vi "setUp.vi"(8 "error in (no error)":errorcluster, 11 "reference in":refnum<class "Disabled Custom Device.lvclass">) -> (0 "error out":errorcluster, 3 "reference out":refnum<class "Disabled Custom Device.lvclass">)   [LabVIEW 2020, in "Disabled Custom Device.lvclass"]
doc: "setUp runs prior to the test method during test execution. Use this method to initialize any object data required by your tests."
uses:
  Disabled Custom Device.lvclass
  C:/Program Files (x86)/National Instruments/LabVIEW 2020/vi.lib/addons/_JKI Toolkits/VI Tester/TestCase.llb/TestCase.lvclass
  Disabled Custom Device.lvclass/Disabled Custom Device.ctl
  <vilib>/addons/_JKI Toolkits/VI Tester/TestCase.llb/TestCase.lvclass
  niveristand-custom-device-testing-tools/VeriStandTestUtilities/VeriStandTestUtilities.lvlib
  Scripting/Ballard/Ballard ARINC 429 Scripting.lvlib
  C:/dev/git/niveristand-custom-device-testing-tools/VeriStandTestCase/VeriStandTestCase.lvclass
  C:/dev/git/niveristand-ballard-arinc429-custom-device/Source/Custom Device Support/Tests/System/Disabled Custom Device/Disabled Custom Device.lvclass
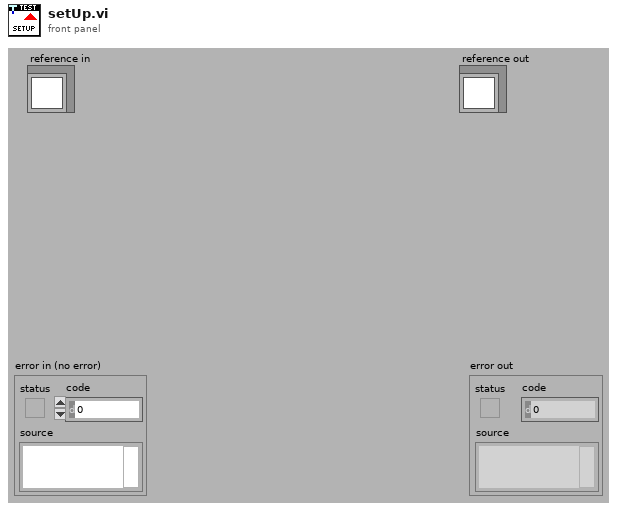
[diagram p1: front panel]
types:
  T1 = typedef "Custom Device API.lvlib/Custom Device Item Ref.ctl" = u64
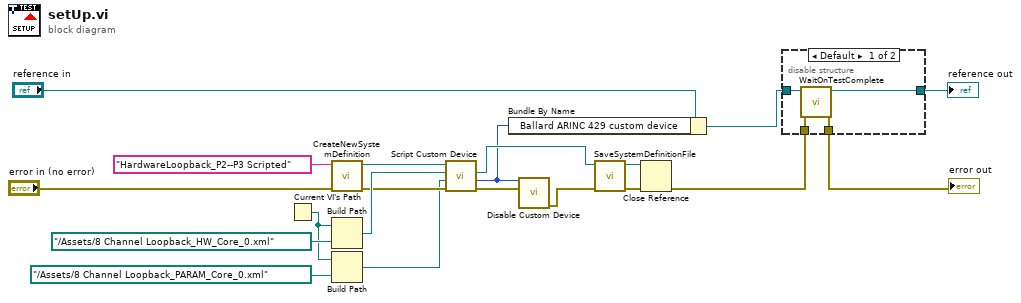
[diagram p0: block diagram]
diagram:
  n1 = Current VI's Path() -> (path=w4:path)
  n2 = call "CreateNewSystemDefinition.vi"("error in"="error in (no error)", "System Definition Name"="HardwareLoopback_P2--P3 Scripted" ("Channel")) -> ("error out"=w13:errorcluster, "System Definition Path"=w12:path)  [unwired: 8 in]
  n3 = Build Path(base path=w4, name or relative path=path "../Assets/8 Channel Loopback_HW_Core_0.xml" ("Hardware File Path")) -> (appended path=w17:path)
  n4 = Build Path(base path=w4, name or relative path=path "../Assets/8 Channel Loopback_PARAM_Core_0.xml" ("Hardware File Path")) -> (appended path=w5:path)
  n5 = call "Script Custom Device.vi"("error in"=w13, "Parameter File Path"=w5, "Hardware File Path"=w17, "System Definition File Path In"=w12) -> ("error out"=w3:errorcluster, "Ballard ARINC 429 custom device out"=w1:T1, "System Definition Reference"=w11:refnum<k24>)  [unwired: 4 in, 1 out]
  n6 = Bundle By Name(cluster="reference in", "Ballard ARINC 429 custom device"=w1) -> (w7:refnum<class "Disabled Custom Device.lvclass">)
  n7 = call "Disable Custom Device.vi"("error in (no error)"=w3, "Ballard ARINC 429 ref"=w1) -> ("error out"=w2:errorcluster)  [unwired: 8 in, 1 out]
  n8 = call "SaveSystemDefinitionFile.vi"("error in (no error)"=w2, "System Definition Reference in"=w11) -> ("error out"=w9:errorcluster, "System Definition Reference out"=w8:refnum<k24>)  [unwired: 8 in]
  n9 = Close Reference(reference=w8, error in (no error)=w9) -> (error out=w6:errorcluster)
  n10 = disable-structure shown="Default" {
    disable-tunnel: w6 -> [w24 w25]
    disable-tunnel: [w23 w25] -> w20
    disable-tunnel: [w22 w26] -> w18
    disable-tunnel: w7 -> [w21 w26]
    frame condition #0 (active) {
      n11 = call <vilib>:"WaitOnTestComplete.vi"("error in (no error)"=w24, "TestCase in"=w21) -> ("error out"=w23:errorcluster, "TestCase out"=w22:refnum<class "Disabled Custom Device.lvclass">)  [unwired: 8 in]
    }
    frame condition #1 {
    }
  }
  "error out" <- w20
  "reference out" <- w18
